vi "NodeMenuActivation.vi"(8 "error in (no error)":errorcluster, 10 "Node Path":string, 11 "xceRootNode in":refnum<class "xceRootNode.lvclass">) -> (0 "error out":errorcluster, 2 "flatMenu[]":T1, 3 "xceRootNode out":refnum<class "xceRootNode.lvclass">)   [LabVIEW 2013, in "xceRootNode.lvclass"]
doc: "Determines the menu options that will be passed to the tree control, after the user activate a menu on the tree control."
uses:
  xceRootNode.lvclass
  _shared/flatMenu.ctl
  xceDataNode/xceDataNode.lvclass
  xceNode/xceNode.lvclass
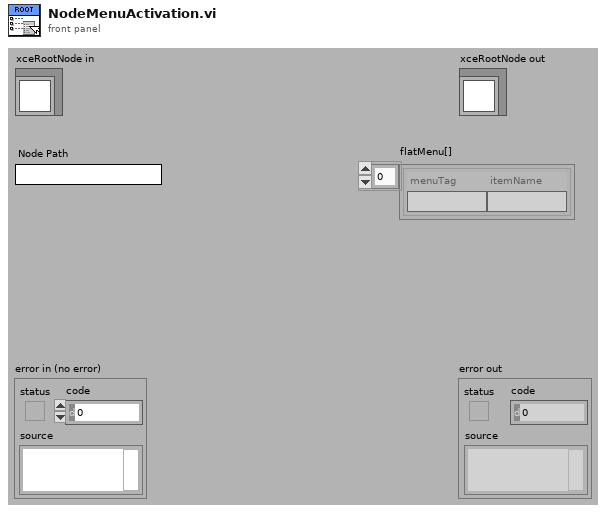
[diagram p1: front panel]
types:
  T1 = typedef "flatMenu.ctl" = cluster{"menuTag":string, "itemName":string}[]
  T2 = cluster{"className":string, "classAlias":string}[]
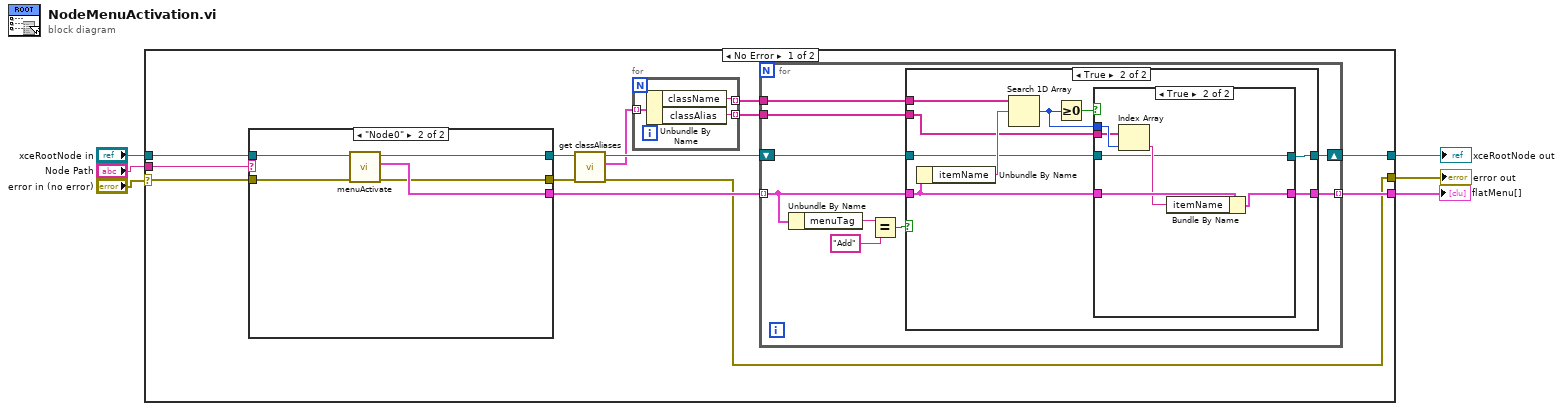
[diagram p0: block diagram]
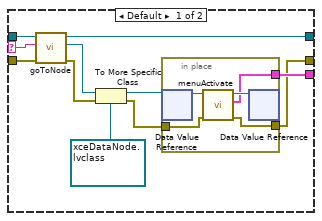
[diagram p4: hidden frame]
diagram:
  n1 = case shown="No Error" "error in (no error)" {
    selector: "error in (no error)" -> [w17 w73]
    tunnel: [w7 w73] -> w5
    tunnel: [w9 w72] -> w3
    tunnel: "xceRootNode in" -> [w19 w72]
    tunnel: "Node Path" -> [w18 _]
    tunnel: [w10 _] -> w1
    frame No Error {
      n2 = case shown="\"Node0\"" w18 {
        selector: w18 -> [w58 _]
        tunnel: w19 -> [w61 w71]
        tunnel: [w60 w70] -> w16
        tunnel: [w52 w69] -> w8
        tunnel: w17 -> [w55 w68]
        tunnel: [w51 w67] -> w15
        frame Default {
          n3 = call "goToNode.vi"("error in (no error)"=w55, "Node Path"=w58, "xceNode in"=w61) -> ("error out"=w54:errorcluster, "goToNode* out"=w59:refnum<data-value>, "xceNode out"=w60:refnum<class "xceRootNode.lvclass">)  [unwired: 6 in]
          n4 = To More Specific Class(target class=refnum<data-value> refnum ("data value reference"), reference=w59, error in=w54) -> (specific class reference=w56:refnum<data-value>, error out=w53:errorcluster)
          n5 = in-place {
            in-place-border: w53 -> [w64]
            in-place-border: [w63] -> w51
            in-place-border: [w62] -> w52
            n6 = in-place-dvr #1(w56) -> (w66:refnum<class "xceDataNode.lvclass">)  [unwired: 1 out]
            n7 = call-dynamic "menuActivate.vi"("error in (no error)"=w64, "xceDataNode in"=w66) -> ("error out"=w63:errorcluster, "flatMenu[] out"=w62:T1, "xceDataNode out"=w65:refnum<class "xceDataNode.lvclass">)  [unwired: 7 in]
            n8 = in-place-dvr #1(w65) -> ()  [unwired: 2 out]
          }
        }
        frame "Node0" {
          n9 = call-dynamic "menuActivate.vi"("error in (no error)"=w68, "xceDataNode in"=w71) -> ("error out"=w67:errorcluster, "flatMenu[] out"=w69:T1, "xceDataNode out"=w70:refnum<class "xceRootNode.lvclass">)  [unwired: 7 in]
        }
      }
      n10 = call "get classAliases.vi"("error in (no error)"=w15, "xceRootNode in"=w16) -> ("error out"=w7:errorcluster, "classAliases"=w13:T2, "xceRootNode out"=w14:refnum<class "xceRootNode.lvclass">)  [unwired: 7 in]
      n11 = for {
        tunnel: w13 -> [w22] mode=indexing
        tunnel: [w21] -> w12 mode=indexing
        tunnel: [w20] -> w11 mode=indexing
        n12 = Unbundle By Name(w22) -> ("className"=w21:string, "classAlias"=w20:string)
      }
      n13 = for {
        tunnel: w8 -> [w29] mode=indexing
        tunnel: w12 -> [w27]
        tunnel: w11 -> [w26]
        tunnel: [w25] -> w10 mode=indexing
        shift-right: [w23] -> w9
        shift-left: w14 -> [w28]
        n14 = Unbundle By Name(w29) -> ("menuTag"=w31:string)
        n15 = Equal?(x=w31, y="Add") -> (x = y?=w24:bool)
        n16 = case shown="True" w24 {
          tunnel: w29 -> [w33 w39]
          tunnel: w28 -> [w32 w35]
          tunnel: w27 -> [_ w42]
          tunnel: w26 -> [_ w38]
          tunnel: [w33 w36] -> w25
          tunnel: [w32 w34] -> w23
          frame False {
          }
          frame True {
            n17 = Unbundle By Name(w39) -> ("itemName"=w41:string)
            n18 = Search 1D Array(1D array=w42, element=w41) -> (index of element=w37:i32)  [unwired: 1 in]
            n19 = Greater Or Equal To 0?(x=w37) -> (x >= 0?=w40:bool)
            n20 = case shown="True" w40 {
              tunnel: w39 -> [w44 w50]
              tunnel: w38 -> [_ w48]
              tunnel: w37 -> [_ w49]
              tunnel: [w44 w46] -> w36
              tunnel: w35 -> [w43 w45]
              tunnel: [w43 w45] -> w34
              frame False {
              }
              frame True {
                n21 = Index Array(array=w48, index=w49) -> (element=w47:string)
                n22 = Bundle By Name(cluster=w50, "itemName"=w47) -> (w46:cluster{"menuTag":string, "itemName":string})
              }
            }
          }
        }
      }
    }
    frame Error {
    }
  }
  "error out" <- w5
  "xceRootNode out" <- w3
  "flatMenu[]" <- w1
